vi "setSerializedData.vi"(0 "reference":refnum<class "ImplicitParameterNode.lvclass">, 1 "parent":refnum<class "AbstractNode.lvclass">, 2 "children":refnum<class "AbstractNode.lvclass">[](array[class]), 3 "xmlOut":string, 5 "error in (no error)":errorcluster) -> (14 "reference out":refnum<class "ImplicitParameterNode.lvclass">, 19 "error out":errorcluster)   [LabVIEW 2014, in "ImplicitParameterNode.lvclass"]
doc: "setSerializedData"
uses:
  <resource>/Framework/Providers/Open_GDS/UML/ImplicitParameterNode_class/ImplicitParameterNode.lvclass
  <resource>/Framework/Providers/Open_GDS/UML/AbstractNode_class/AbstractNode.lvclass
  <resource>/Framework/Providers/Open_GDS/UML/AbstractNode_class/ObjectReference.ctl
  <resource>/Framework/Providers/Open_GDS/UML/General/Rectangle/Rectangle Rectangle2D.ctl
  <resource>/Framework/Providers/Open_GDS/UML/MultiLineString_class/ObjectReference.ctl
  <resource>/Framework/Providers/Open_GDS/UML/MultiLineString_class/MultiLineString.lvclass
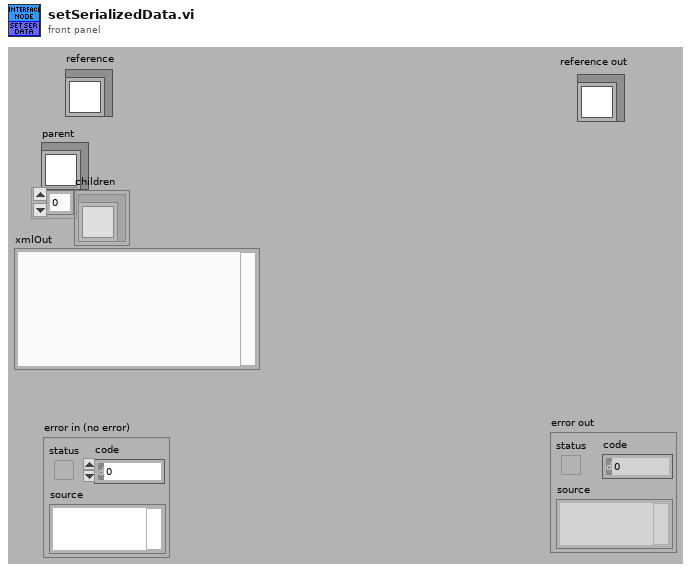
[diagram p1: front panel]
types:
  T1 = typedef "AbstractNode.lvclass/ObjectReference.ctl" = refnum<k1>
  T2 = typedef "Rectangle Rectangle2D.ctl" = cluster{"x":dbl, "y":dbl, "width":dbl, "height":dbl}
  T3 = typedef "MultiLineString.lvclass/ObjectReference.ctl" = refnum<k1>
  T4 = cluster{"Base class":cluster{"Base class":cluster{"parent":T1, "children":T1[]}, "bounds":T2}, "topHeight":dbl, "name":T3, "DEFAULT_TOP_HEIGHT":i32, "DEFAULT_WIDTH":i32, "DEFAULT_HEIGHT":i32}
  T5 = typedef "ImplicitParameterNode.lvclass/ObjectAttributes.ctl" = cluster{"Base class":T6, "topHeight":dbl, "name":refnum<class "MultiLineString.lvclass">, "DEFAULT_TOP_HEIGHT":i32, "DEFAULT_WIDTH":i32, "DEFAULT_HEIGHT":i32}
  T6 = typedef "RectangularNode.lvclass/ObjectAttributes.ctl" = cluster{"Base class":T7, "bounds":T2}
  T7 = typedef "AbstractNode.lvclass/ObjectAttributes.ctl" = cluster{"parent":refnum<class "AbstractNode.lvclass">, "children":refnum<class "AbstractNode.lvclass">[], "Hidden":bool}
  T8 = cluster{"Attributes":cluster{"Base class":cluster{"Base class":cluster{"parent":T1, "children":T1[]}, "bounds":T2}, "topHeight":dbl, "name":T3, "DEFAULT_TOP_HEIGHT":i32, "DEFAULT_WIDTH":i32, "DEFAULT_HEIGHT":i32}, string}
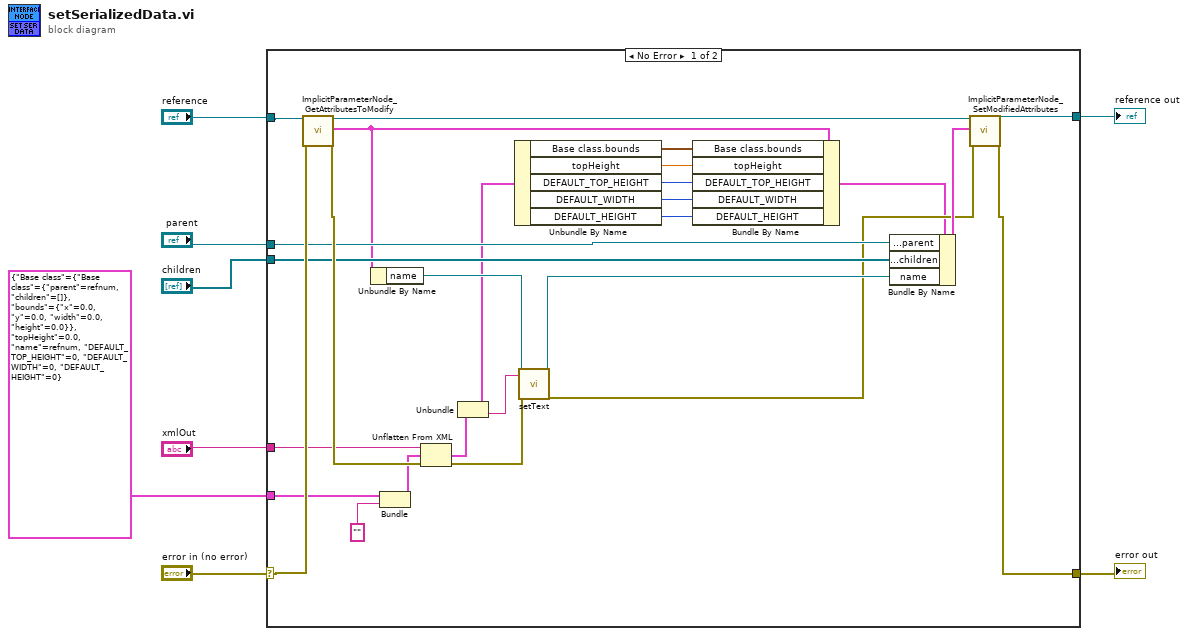
[diagram p0: block diagram]
diagram:
  n1 = case shown="No Error" "error in (no error)" {
    selector: "error in (no error)" -> [w25 w36]
    tunnel: "reference" -> [w26 w37]
    tunnel: [w24 w36] -> w6
    tunnel: [w22 w37] -> w5
    tunnel: "xmlOut" -> [w23 _]
    tunnel: "parent" -> [w21 _]
    tunnel: "children" -> [w20 _]
    tunnel: T4 {"Base class"={"Base class"={"parent"=refnum, "children"=[]}, "bounds"={"x"=0.0, "y"=0.0, "width"=0.0, "height"=0.0}}, "topHeight"=0.0, "name"=refnum, "DEFAULT_TOP_HEIGHT"=0, "DEFAULT_WIDTH"=0, "DEFAULT_HEIGHT"=0} ("Attributes") -> [w17 _]
    frame No Error {
      n2 = call <resource>:"ImplicitParameterNode_GetAttributesToModify.vi"("reference in"=w26, "error in (no error)"=w25) -> ("reference out"=w35:refnum<class "ImplicitParameterNode.lvclass">, "Attributes"=w10:T5, "error out"=w33:errorcluster)  [unwired: 1 in, 14 out]
      n3 = Unbundle By Name(w10) -> ("name"=w32:refnum<class "MultiLineString.lvclass">)
      n4 = Bundle("Attributes"=w17, "") -> (w31:T8)  [unwired: 1 out]
      n5 = Unflatten From XML(xml string=w23, type=w31, error in (no error)=w33) -> (value=w28:T8, error out=w30:errorcluster)
      n6 = Unbundle(w28) -> ("Attributes"=w11:T4, w27:string)
      n7 = Unbundle By Name(w11) -> ("Base class.bounds"=w16:T2, "topHeight"=w15:dbl, "DEFAULT_TOP_HEIGHT"=w14:i32, "DEFAULT_WIDTH"=w13:i32, "DEFAULT_HEIGHT"=w12:i32)
      n8 = call-dynamic "setText.vi"("reference"=w32, "text"=w27, "error in (no error)"=w30) -> ("reference out"=w29:refnum<class "MultiLineString.lvclass">, "error out"=w19:errorcluster)  [unwired: 15 out]
      n9 = Bundle By Name(cluster=w10, "Base class.bounds"=w16, "topHeight"=w15, "DEFAULT_TOP_HEIGHT"=w14, "DEFAULT_WIDTH"=w13, "DEFAULT_HEIGHT"=w12) -> (w9:T5)
      n10 = Bundle By Name(cluster=w9, "Base class.Base class.parent"=w21, "Base class.Base class.children"=w20, "name"=w29) -> (w34:T5)
      n11 = call <resource>:"ImplicitParameterNode_SetModifiedAttributes.vi"("reference in"=w35, "Attributes"=w34, "error in (no error)"=w19) -> ("reference out"=w22:refnum<class "ImplicitParameterNode.lvclass">, "error out"=w24:errorcluster)  [unwired: 3 in, 12 out]
    }
    frame Error {
    }
  }
  "reference out" <- w5
  "error out" <- w6
